vi "Plotmatrix Scale Property.vi"(4 "Max Range":T1, 6 "Update?":bool, 8 "error in (no error)":errorcluster, 9 "Scale Array In":T2, 11 "Single XY Plot In":refnum<vi>) -> (0 "error out":errorcluster, 1 "Scale Array Out":T2, 3 "Single XY Plot Out":refnum<vi>)   [LabVIEW 2020, in "XY Plot Matrix.lvclass"]
uses:
  <vilib>/Math Plots/2D Math Plots/XY Plot Matrix/XY Plot Matrix/XY Plot Matrix.lvclass
  <vilib>/Math Plots/2D Math Plots/2D Plot/2D Plot/Typedef/Scale Array.ctl
  <vilib>/Math Plots/2D Math Plots/2D Plot/2D Plot/Typedef/Scale Cluster.ctl
  <vilib>/Utility/miscctls.llb/LVOffsetAndMultiplierTypeDef.ctl
  <vilib>/Math Plots/2D Math Plots/2D Plot/2D Plot/Typedef/Range Cluster.ctl
  <vilib>/Math Plots/2D Math Plots/2D Plot/2D Plot/2D Plot.lvclass
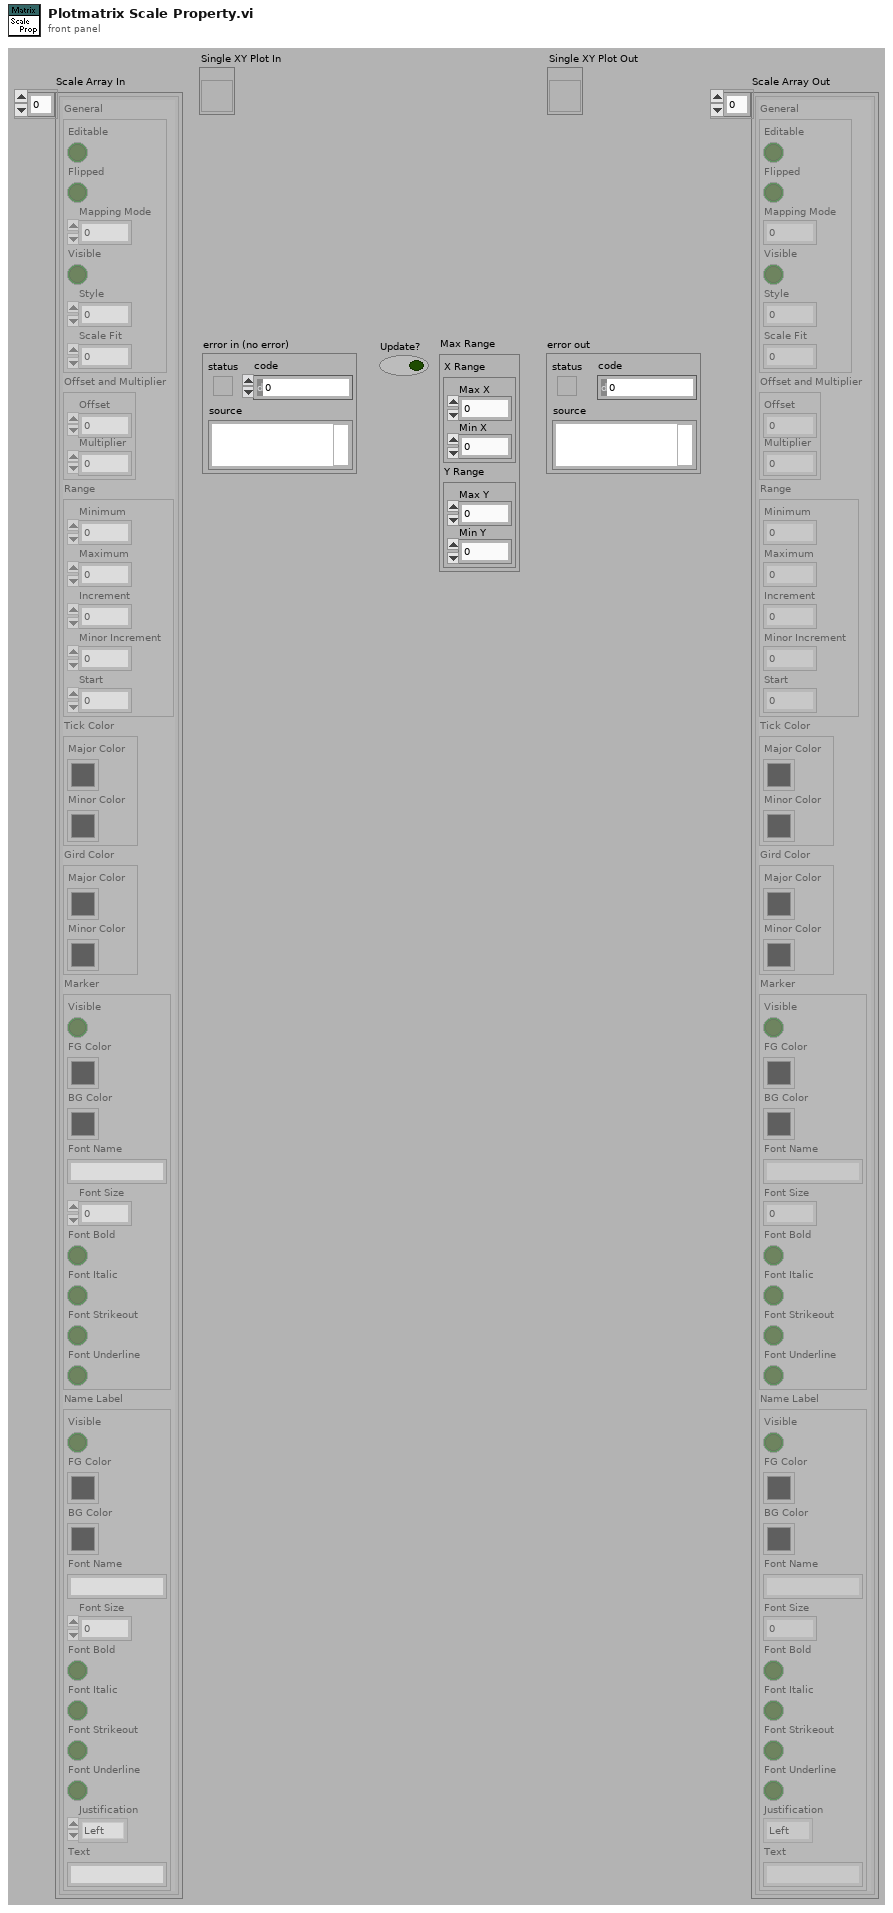
[diagram p1: front panel]
types:
  T1 = typedef "2D Plot.lvclass/Range Cluster.ctl" = cluster{"X Range":cluster{"Max X":dbl, "Min X":dbl}, "Y Range":cluster{"Max Y":dbl, "Min Y":dbl}}
  T2 = typedef "2D Plot.lvclass/Scale Array.ctl" = T3[]
  T3 = typedef "2D Plot.lvclass/Scale Cluster.ctl" = cluster{"General":cluster{"Editable":bool, "Flipped":bool, "Mapping Mode":u8, "Visible":bool, "Style":u8, "Scale Fit":u8}, "Offset and Multiplier":T4, "Range":cluster{"Minimum":dbl, "Maximum":dbl, "Increment":dbl, "Minor Increment":dbl, "Start":dbl}, "Tick Color":cluster{"Major Color":u32, "Minor Color":u32}, "Gird Color":cluster{"Major Color":u32, "Minor Color":u32}, "Marker":cluster{"Visible":bool, "FG Color":u32, "BG Color":u32, "Font Name":string, "Font Size":u32, "Font Bold":bool, "Font Italic":bool, "Font Strikeout":bool, "Font Underline":bool}, "Name Label":cluster{"Visible":bool, "FG Color":u32, "BG Color":u32, "Font Name":string, "Font Size":u32, "Font Bold":bool, "Font Italic":bool, "Font Strikeout":bool, "Font Underline":bool, "Justification":enum16{"Left", "Center", "Right"}, "Text":string}}
  T4 = typedef "LVOffsetAndMultiplierTypeDef.ctl" = cluster{"Offset":dbl, "Multiplier":dbl}
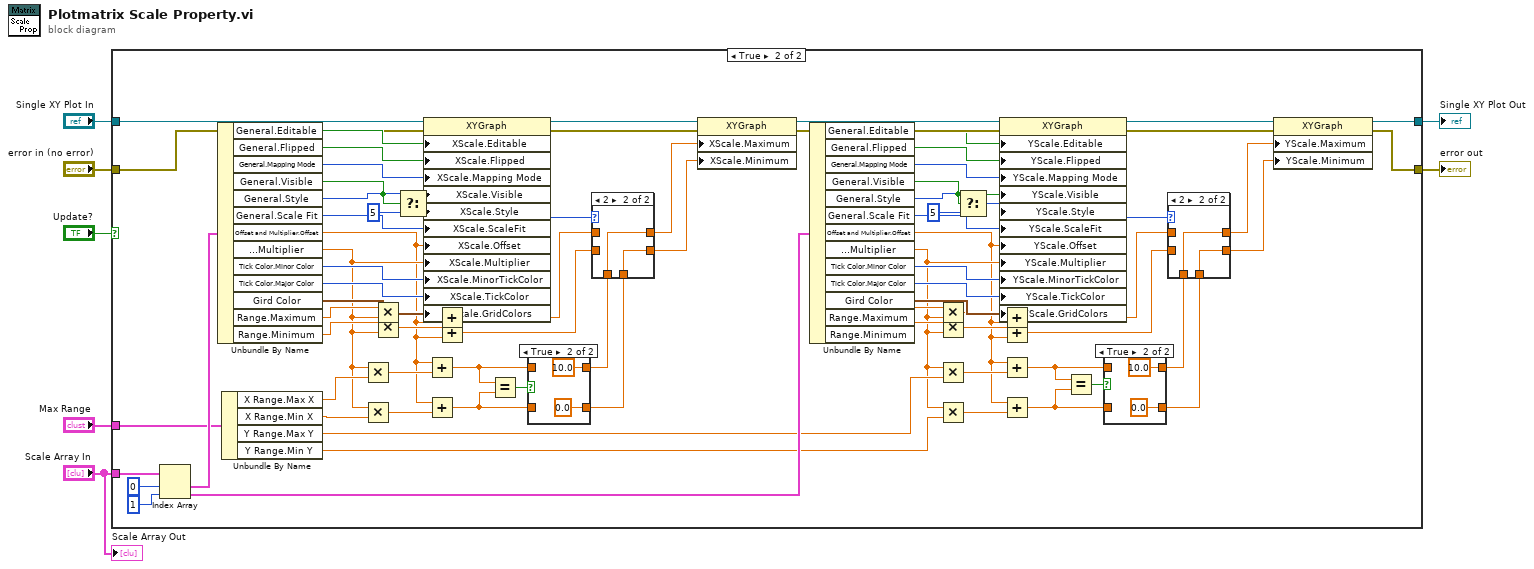
[diagram p0: block diagram]
diagram:
  n1 = case shown="True" "Update?" {
    tunnel: "Single XY Plot In" -> [w9 w57]
    tunnel: "error in (no error)" -> [w8 w56]
    tunnel: [w9 w55] -> w5
    tunnel: [w8 w54] -> w4
    tunnel: "Scale Array In" -> [_ w53]
    tunnel: "Max Range" -> [_ w50]
    frame False {
    }
    frame True {
      n2 = Index Array(array=w53, index #1=0 ("index"), index #2=1 ("index")) -> (element #1=w59:T3, element #2=w58:T3)
      n3 = Unbundle By Name(w59) -> ("General.Editable"=w70:bool, "General.Flipped"=w60:bool, "General.Mapping Mode"=w61:u8, "General.Visible"=w73:bool, "General.Style"=w74:u8, "General.Scale Fit"=w27:u8, "Offset and Multiplier.Offset"=w28:dbl, "Offset and Multiplier.Multiplier"=w30:dbl, "Tick Color.Minor Color"=w62:u32, "Tick Color.Major Color"=w68:u32, "Gird Color"=w63:cluster{"Major Color":u32, "Minor Color":u32}, "Range.Maximum"=w35:dbl, "Range.Minimum"=w31:dbl)
      n4 = Unbundle By Name(w50) -> ("X Range.Max X"=w49:dbl, "X Range.Min X"=w44:dbl, "Y Range.Max Y"=w43:dbl, "Y Range.Min Y"=w42:dbl)
      n5 = Multiply(x=w30, y=w49) -> (x*y=w47:dbl)
      n6 = Multiply(x=w30, y=w44) -> (x*y=w48:dbl)
      n7 = Multiply(x=w35, y=w30) -> (x*y=w32:dbl)
      n8 = Multiply(x=w31, y=w30) -> (x*y=w29:dbl)
      n9 = Select(t=w74, s=w73, f=u8 5) -> (s? t:f=w75:u8)
      n10 = property class="XYGraph"(reference=w57, error in=w56, "XScale.Editable"=w70, "XScale.Flipped"=w60, "XScale.Mapping Mode"=w61, "XScale.Visible"=w73, "XScale.Style"=w75, "XScale.ScaleFit"=w27, "XScale.Offset"=w28, "XScale.Multiplier"=w30, "XScale.MinorTickColor"=w62, "XScale.TickColor"=w68, "XScale.GridColors"=w63) -> (reference out=w80:refnum<vi>, error out=w81:errorcluster)
      n11 = Add(x=w28, y=w47) -> (x+y=w40:dbl)
      n12 = Add(x=w28, y=w48) -> (x+y=w39:dbl)
      n13 = Add(x=w32, y=w28) -> (x+y=w22:dbl)
      n14 = Add(x=w29, y=w28) -> (x+y=w21:dbl)
      n15 = Equal?(x=w40, y=w39) -> (x = y?=w41:bool)
      n16 = case shown="True" w41 {
        tunnel: [w99 10.0] -> w26
        tunnel: w40 -> [w99 _]
        tunnel: [w98 0.0] -> w25
        tunnel: w39 -> [w98 _]
        frame False {
        }
        frame True {
        }
      }
      n17 = case shown="2" w27 {
        tunnel: w26 -> [_ w93]
        tunnel: w25 -> [_ w92]
        tunnel: [w91 w93] -> w24
        tunnel: [w90 w92] -> w23
        tunnel: w22 -> [w91 _]
        tunnel: w21 -> [w90 _]
        frame Default {
        }
        frame 2 {
        }
      }
      n18 = property class="XYGraph"(reference=w80, error in=w81, "XScale.Maximum"=w24, "XScale.Minimum"=w23) -> (reference out=w83:refnum<vi>, error out=w82:errorcluster)
      n19 = Unbundle By Name(w58) -> ("General.Editable"=w71:bool, "General.Flipped"=w64:bool, "General.Mapping Mode"=w65:u8, "General.Visible"=w79:bool, "General.Style"=w77:u8, "General.Scale Fit"=w16:u8, "Offset and Multiplier.Offset"=w17:dbl, "Offset and Multiplier.Multiplier"=w18:dbl, "Tick Color.Minor Color"=w66:u32, "Tick Color.Major Color"=w69:u32, "Gird Color"=w67:cluster{"Major Color":u32, "Minor Color":u32}, "Range.Maximum"=w33:dbl, "Range.Minimum"=w19:dbl)
      n20 = Multiply(x=w33, y=w18) -> (x*y=w34:dbl)
      n21 = Multiply(x=w19, y=w18) -> (x*y=w20:dbl)
      n22 = Multiply(x=w18, y=w43) -> (x*y=w45:dbl)
      n23 = Multiply(x=w18, y=w42) -> (x*y=w46:dbl)
      n24 = Select(t=w77, s=w79, f=u8 5) -> (s? t:f=w78:u8)
      n25 = property class="XYGraph"(reference=w83, error in=w82, "YScale.Editable"=w71, "YScale.Flipped"=w64, "YScale.Mapping Mode"=w65, "YScale.Visible"=w79, "YScale.Style"=w78, "YScale.ScaleFit"=w16, "YScale.Offset"=w17, "YScale.Multiplier"=w18, "YScale.MinorTickColor"=w66, "YScale.TickColor"=w69, "YScale.GridColors"=w67) -> (reference out=w84:refnum<vi>, error out=w85:errorcluster)
      n26 = Add(x=w34, y=w17) -> (x+y=w15:dbl)
      n27 = Add(x=w20, y=w17) -> (x+y=w14:dbl)
      n28 = Add(x=w17, y=w45) -> (x+y=w37:dbl)
      n29 = Add(x=w17, y=w46) -> (x+y=w36:dbl)
      n30 = Equal?(x=w37, y=w36) -> (x = y?=w38:bool)
      n31 = case shown="True" w38 {
        tunnel: [w95 10.0] -> w13
        tunnel: w37 -> [w95 _]
        tunnel: [w94 0.0] -> w12
        tunnel: w36 -> [w94 _]
        frame False {
        }
        frame True {
        }
      }
      n32 = case shown="2" w16 {
        tunnel: w13 -> [_ w89]
        tunnel: w12 -> [_ w88]
        tunnel: [w87 w89] -> w11
        tunnel: [w86 w88] -> w10
        tunnel: w15 -> [w87 _]
        tunnel: w14 -> [w86 _]
        frame Default {
        }
        frame 2 {
        }
      }
      n33 = property class="XYGraph"(reference=w84, error in=w85, "YScale.Maximum"=w11, "YScale.Minimum"=w10) -> (reference out=w55:refnum<vi>, error out=w54:errorcluster)
    }
  }
  "Single XY Plot Out" <- w5
  "error out" <- w4
  "Scale Array Out" <- "Scale Array In"
